vi "Generate Model Updated.vi"(0 "Resonance Frequency [Hz]":dbl, 1 "Drive Frequency [Hz]":dbl, 2 "Q Factor":dbl, 3 "Sampling Time [us]":u8, 4 "L1":dbl, 5 "L2":dbl, 6 "k":dbl=1.0) -> (9 "error out":errorcluster)   [LabVIEW 2013]
uses:
  <vilib>/addons/Control Design/_Model Construction/Model Typedefs.llb/CD State Space Model (MIMO).ctl
  <vilib>/addons/Control Design/_Model Construction/Model Typedefs.llb/CD General Elements.ctl
  <vilib>/Analysis/Matrix/Datatypes/RealMatrix.ctl
  <vilib>/Analysis/baseanly.llb/Real A x B.vi
  <vilib>/Analysis/7linalg.llb/Real Matrix Power.vi
  <vilib>/Analysis/7linalg.llb/Real Transpose Matrix.vi
  <vilib>/Analysis/Matrix/Numeric/Conversions/Array To Matrix - RA.vi
  <vilib>/addons/Control Design/_Model Construction/Model Creation.llb/Model Creation SubVI/cd_Create State Space Model.vi
  <vilib>/addons/Control Design/_Model Conversions/Continuous and Discrete.llb/Continuous and Discrete SubVI/cd_Convert Continuous to Discrete (SS).vi
  <vilib>/Analysis/Matrix/Numeric/Conversions/Array To Matrix - RA2.vi
  <vilib>/Analysis/Matrix/Numeric/Subtract/Subtract - RM,RM.vi
  <vilib>/Analysis/baseanly.llb/Real Inverse Matrix.vi
  <vilib>/Analysis/Matrix/Numeric/Conversions/Matrix To Array - RM.vi
  <vilib>/addons/Control Design/_Model Construction/NI_LinSys_Model Creation.lvlib
  <vilib>/addons/Control Design/_Model Conversions/NI_CD_Continuous and Discrete.lvlib
  <vilib>/Analysis/Matrix/NI_Matrix.lvlib
  <vilib>/Analysis/NI_AALBase.lvlib
  <vilib>/Analysis/NI_AALPro.lvlib
  <vilib>/addons/Control Design/_Model Construction/NI_LinSys_Model Typedefs.lvlib
panel:
  out "Discrete State-Space Model":T1 {"Transport Delay" format="%.2f"; "D" format="%#.2g"; "C" format="%#.2g"; "B" format="%#.2g"; "A" format="%#.2g"; "properties"."Sampling Time" format="%#.6p"; "properties"."Output Delays" format="%.4f"; "properties"."Input Delays" format="%.4f"}
  out "F":dbl[][](array[numeric])
  out "G":dbl[][](array[numeric])
  out "C":dbl[][](array[numeric])
  in  "V":dbl
  out "(1/V^2)":dbl
  out "Coeff 1":dbl[](array[numeric])
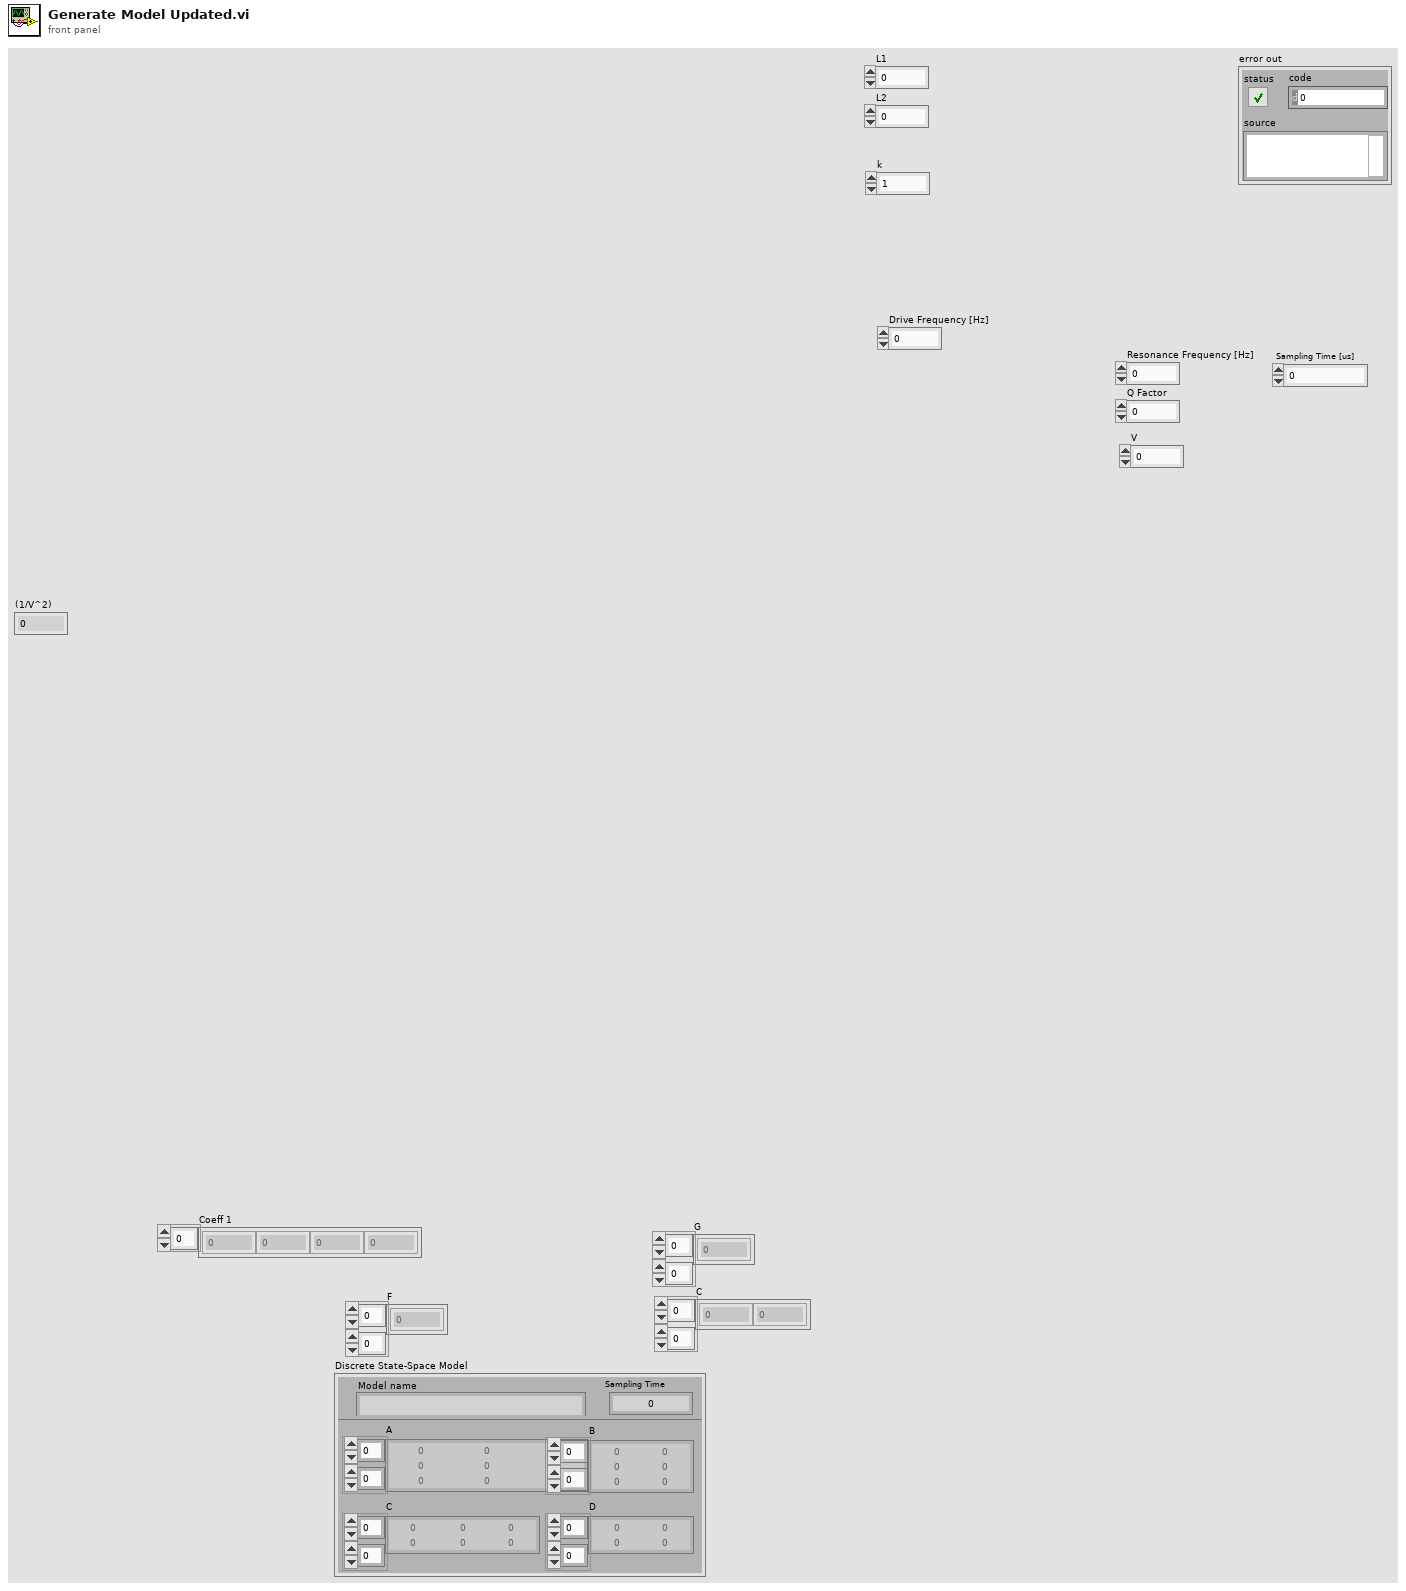
[diagram p1: front panel]
types:
  T1 = typedef "NI_LinSys_Model Typedefs.lvlib/CD State Space Model (MIMO).ctl" = cluster{"properties":T2, "A":dbl[][], "B":dbl[][], "C":dbl[][], "D":dbl[][], "StateNames":string[], "Transport Delay":dbl[][]}
  T2 = typedef "NI_LinSys_Model Typedefs.lvlib/CD General Elements.ctl" = cluster{"Model name":string, "Input names":string[], "Output names":string[], "Input Delays":dbl[], "Output Delays":dbl[], "Sampling Time":dbl, "Notes":string}
  T3 = typedef "NI_Matrix.lvlib/RealMatrix.ctl" = dbl[][]
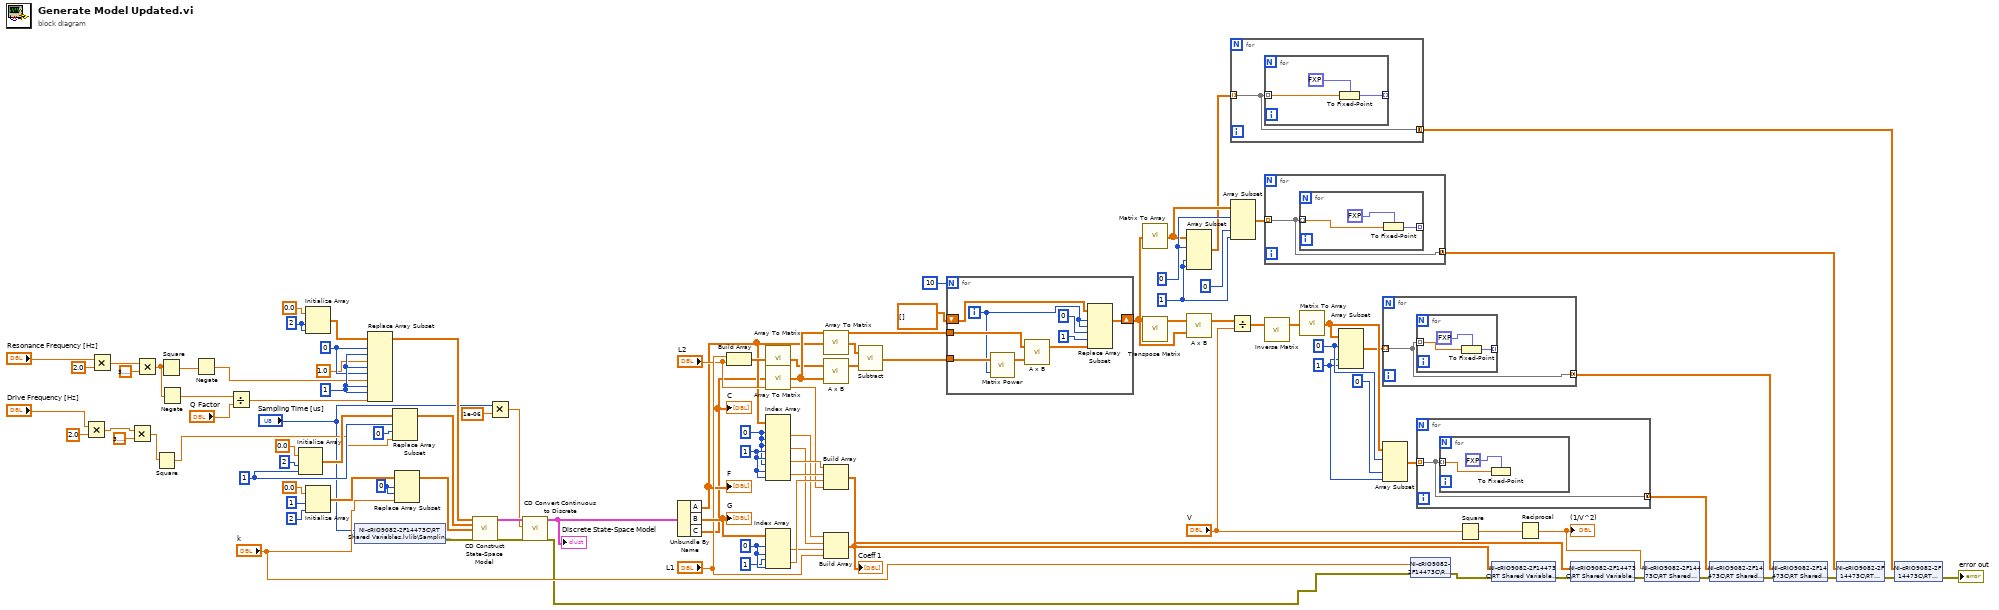
[diagram p0: block diagram]
diagram:
  w32 = 1 ("length")
  w33 = 0 ("index")
  w86 = 1 ("length")
  w85 = 0 ("index")
  w74 = 0 ("index (row)")
  w76 = 1 ("disabled index (col)")
  w75 = 0 ("index (row)")
  w70 = 1 ("dimension size")
  w41 = 0 ("index (row)")
  w57 = 1 ("disabled index (col)")
  w48 = 0 ("index (row)")
  w44 = 2 ("dimension size")
  n1 = Multiply(x="Drive Frequency [Hz]", y=2.0) -> (x*y=w11:dbl)
  n2 = Multiply(x="Resonance Frequency [Hz]", y=2.0) -> (x*y=w52:dbl)
  n3 = Multiply(x=w11, y=3.141592653589793) -> (x*y=w10:dbl)
  n4 = Multiply(x=w52, y=3.141592653589793) -> (x*y=w54:dbl)
  n5 = Square(x=w10) -> (x^2=w9:dbl)
  n6 = Square(x=w54) -> (x^2=w15:dbl)
  n7 = Negate(x=w54) -> (-x=w55:dbl)
  n8 = Negate(x=w15) -> (-x=w49:dbl)
  n9 = Divide(x=w55, y="Q Factor") -> (x/y=w58:dbl)
  n10 = Initialize Array(0.0 ("element"), 2 ("dimension size"), w70) -> (w67:dbl[][])
  n11 = Initialize Array(0.0 ("element"), w44, w44) -> (w46:dbl[][])
  n12 = Initialize Array(0.0 ("element"), 1 ("dimension size"), 2 ("dimension size")) -> (w63:dbl[][])
  n13 = shared-variable "NI-cRIO9082-2F14473C\\RT Shared Variables.lvlib\\Sampling Rate"("Sampling Time [us]") -> (error out=w24:errorcluster)  [unwired: 1 in]
  n14 = Replace Array Subset(array=w46, new element #1=1.0 ("element"), index (row) #1=w48, index (col) #1=w57, new element #2=w49, index (row) #2=w57, index (col) #2=w48, new element #3=w58, index (row) #3=w57, index (col) #3=w57) -> (w59:dbl[][])
  n15 = Replace Array Subset(array=w67, new element=w9, index (row)=w70, index (col)=0 ("index (row)")) -> (w71:dbl[][])
  n16 = Replace Array Subset(array=w63, new element="k", index (row)=w41, index (col)=w41) -> (w65:dbl[][])
  n17 = call-poly <vilib>:"CD Construct State-Space Model.vi"("A"=w59, "B"=w71, "C"=w65, "error in (no error)"=w24) -> ("State-Space Model"=w72:T1, "error out"=w23:errorcluster)  [unwired: 10 in]
  n18 = Multiply(x="Sampling Time [us]", y=1e-06) -> (x*y=w5:dbl)
  n19 = call-poly <vilib>:"CD Convert Continuous to Discrete.vi"("error in (no error)"=w23, "Sampling Time (s)"=w5, "Continuous State-Space Model"=w72) -> ("error out"=w4:errorcluster, "Discrete State-Space Model"=w3:T1)  [unwired: 6 in, 1 out]
  "Discrete State-Space Model" <- w3
  n20 = Unbundle By Name(w3) -> ("A"=w2:dbl[][], "B"=w77:dbl[][], "C"=w1:dbl[][])
  "F" <- w2
  "G" <- w77
  "C" <- w1
  n21 = Build Array("L1", "L2") -> (w78:dbl[])
  n22 = call-poly <vilib>:"Array To Matrix.vi"("Real 1D Array"=w78) -> ("Real Matrix (Column Vector)"=w43:T3)
  n23 = call-poly <vilib>:"Array To Matrix.vi"("Real 2D Array"=w1) -> ("Real Matrix"=w80:T3)
  n24 = Index Array(array=w2, index (row) #1=w75, index (col) #1=w75, index (row) #2=w75, index (col) #2=w76, index (row) #3=w76, index (col) #3=w75, index (row) #4=w76, index (col) #4=w76) -> (element #1=w89:dbl, element #2=w90:dbl, element #3=w92:dbl, element #4=w93:dbl)
  n25 = Index Array(array=w77, index (row) #1=w74, index (col) #1=w74, index (row) #2=1 ("disabled index (col)"), index (col) #2=w74) -> (element #1=w91:dbl, element #2=w94:dbl)
  n26 = call-poly <vilib>:"Array To Matrix.vi"("Real 2D Array"=w2) -> ("Real Matrix"=w79:T3)
  n27 = call-poly <vilib>:"A x B.vi"("B"=w80, "A"=w43) -> ("A x B"=w81:T3)  [unwired: 1 out]
  n28 = Build Array(w92, w93, w94, "L2") -> (w100:dbl[])
  n29 = Build Array(w89, w90, w91, "L1") -> (w99:dbl[])
  "Coeff 1" <- w99
  n30 = call-poly <vilib>:"Subtract.vi"("Real Matrix B"=w81, "Real Matrix A"=w79) -> ("A - B"=w82:T3)
  n31 = for {
    N: 10 -> [_]
    tunnel: w80 -> [w110]
    tunnel: w82 -> [w109]
    shift-right: [w105] -> w38
    shift-left: T3 [] ("matrix") -> [w107]
    i -> [w104]
    n32 = call-poly <vilib>:"Matrix Power.vi"("n"=w104, "Input Matrix"=w109) -> ("Matrix Power"=w108:T3)  [unwired: 1 out]
    n33 = call-poly <vilib>:"A x B.vi"("B"=w108, "A"=w110) -> ("A x B"=w106:T3)  [unwired: 1 out]
    n34 = Replace Array Subset(array=w107, new element=w106, index (dim 0)=w104, index (dim 1)=w104, index (dim 2)=0 ("column 1"), index (dim 3)=1 ("column N")) -> (w105:T3)
  }
  n35 = call-poly <vilib>:"Matrix To Array.vi"("Real Matrix"=w38) -> ("Real 2D Array"=w84:dbl[][])
  n36 = call-poly <vilib>:"Transpose Matrix.vi"("Input Matrix"=w38) -> ("Matrix Transpose"=w39:T3)  [unwired: 9 in, 1 out]
  n37 = Array Subset(array=w84, index (row)=w85, index (col)=w86, length (col)=w86) -> (w40:dbl[][])  [unwired: 1 in]
  n38 = call-poly <vilib>:"A x B.vi"("B"=w38, "A"=w39) -> ("A x B"=w37:T3)  [unwired: 1 out]
  n39 = Divide(x=w37, y="V") -> (x/y=w36:T3)
  n40 = for {
    tunnel: w40 -> [w111] mode=indexing
    tunnel: [w111] -> w98 mode=concatenating
    n41 = for {
      tunnel: w111 -> [w114] mode=indexing
      tunnel: [w112] -> _ mode=indexing
      n42 = To Fixed-Point(fixed-point type=fxp<+/-,51,24> 0.0, number=w114) -> (fixed-point=w112:fxp<+/-,51,24>)
    }
  }
  n43 = Array Subset(array=w84, index (row)=w85, index (col)=0 ("index"), length (col)=w86) -> (w87:dbl[][])  [unwired: 1 in]
  n44 = for {
    tunnel: w87 -> [w115] mode=indexing
    tunnel: [w115] -> w97 mode=concatenating
    n45 = for {
      tunnel: w115 -> [w118] mode=indexing
      tunnel: [w116] -> _ mode=indexing
      n46 = To Fixed-Point(fixed-point type=fxp<+/-,50,3> 0.0, number=w118) -> (fixed-point=w116:fxp<+/-,50,3>)
    }
  }
  n47 = call-poly <vilib>:"Inverse Matrix.vi"("Input Matrix"=w36) -> ("Inverse Matrix"=w31:T3)  [unwired: 1 in, 1 out]
  n48 = call-poly <vilib>:"Matrix To Array.vi"("Real Matrix"=w31) -> ("Real 2D Array"=w34:dbl[][])
  n49 = Array Subset(array=w34, index (row)=w33, index (col)=w32, length (col)=w32) -> (w29:dbl[][])  [unwired: 1 in]
  n50 = for {
    tunnel: w29 -> [w119] mode=indexing
    tunnel: [w119] -> w96 mode=concatenating
    n51 = for {
      tunnel: w119 -> [w122] mode=indexing
      tunnel: [w120] -> _ mode=indexing
      n52 = To Fixed-Point(fixed-point type=fxp<+/-,50,35> 0.0, number=w122) -> (fixed-point=w120:fxp<+/-,50,35>)
    }
  }
  n53 = Array Subset(array=w34, index (row)=w33, index (col)=0 ("index"), length (col)=w32) -> (w30:dbl[][])  [unwired: 1 in]
  n54 = shared-variable "NI-cRIO9082-2F14473C\\RT Shared Variables.lvlib\\k"("k", error in=w4) -> (error out=w8:errorcluster)
  n55 = for {
    tunnel: w30 -> [w123] mode=indexing
    tunnel: [w123] -> w95 mode=concatenating
    n56 = for {
      tunnel: w123 -> [w125] mode=indexing
      n57 = To Fixed-Point(fixed-point type=fxp<+/-,64,5> 0.0, number=w125) -> ()  [unwired: 1 out]
    }
  }
  n58 = Square(x="V") -> (x^2=w27:dbl)
  n59 = shared-variable "NI-cRIO9082-2F14473C\\RT Shared Variables.lvlib\\Coeff 1"(w99, error in=w8) -> (error out=w22:errorcluster)
  n60 = Reciprocal(x=w27) -> (1/x=w101:dbl)
  "(1/V^2)" <- w101
  n61 = shared-variable "NI-cRIO9082-2F14473C\\RT Shared Variables.lvlib\\Coeff 2"(w100, error in=w22) -> (error out=w21:errorcluster)
  n62 = shared-variable "NI-cRIO9082-2F14473C\\RT Shared Variables.lvlib\\1oV2"(w101, error in=w21) -> (error out=w20:errorcluster)
  n63 = shared-variable "NI-cRIO9082-2F14473C\\RT Shared Variables.lvlib\\inv 1"(w95, error in=w20) -> (error out=w19:errorcluster)
  n64 = shared-variable "NI-cRIO9082-2F14473C\\RT Shared Variables.lvlib\\inv 2"(w96, error in=w19) -> (error out=w18:errorcluster)
  n65 = shared-variable "NI-cRIO9082-2F14473C\\RT Shared Variables.lvlib\\Y 1"(w97, error in=w18) -> (error out=w17:errorcluster)
  n66 = shared-variable "NI-cRIO9082-2F14473C\\RT Shared Variables.lvlib\\Y 2"(w98, error in=w17) -> (error out=→"error out":errorcluster)
